vi "Load Tdms Wfm By Index.vi"(8 "error in (no error)":errorcluster, 10 "Read From":i32, 11 "file path":path) -> (0 "error out":errorcluster, 3 "Waveform":waveform(dbl)(graph))   [LabVIEW 2025, in "TDMS Waveform Creator.lvclass"]
uses:
  TDMS Waveform Creator.lvclass
  TDMS Waveform Creator.lvclass/TDMS Waveform Creator.ctl
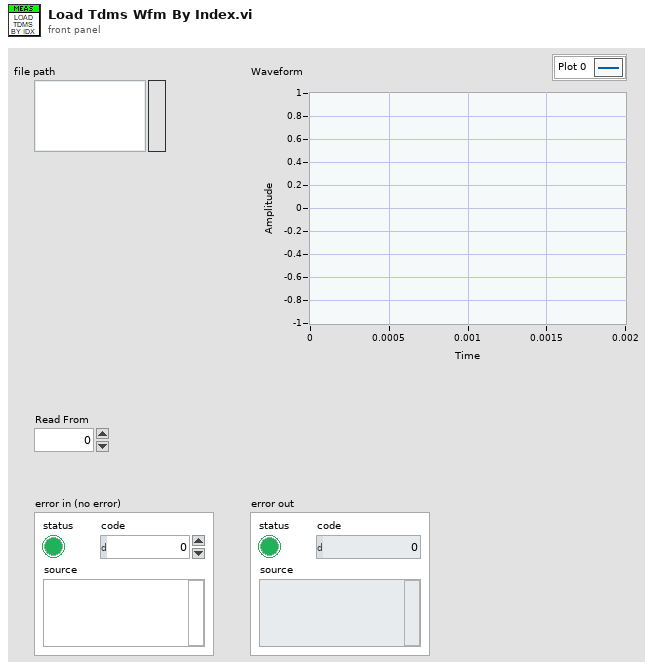
[diagram p1: front panel]
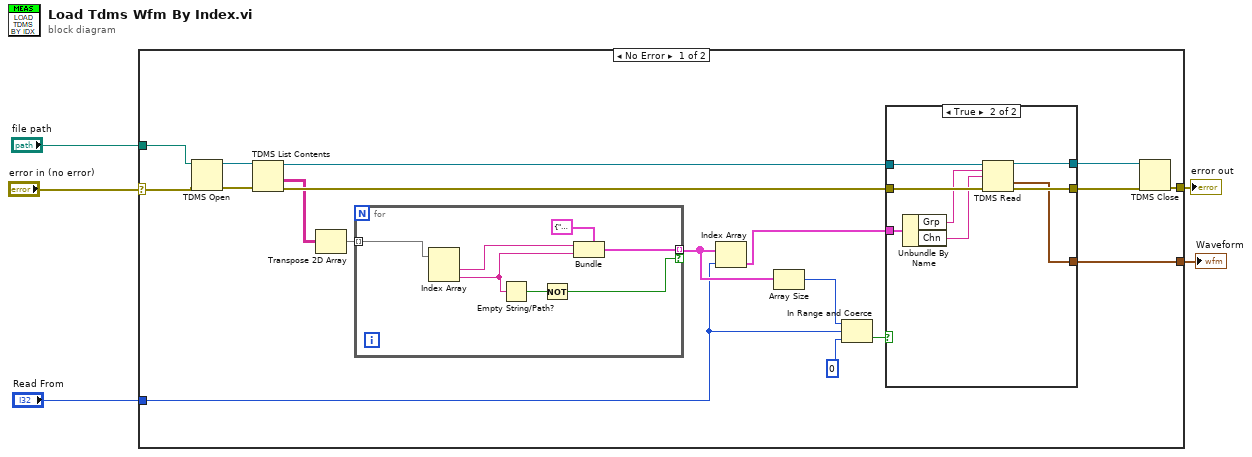
[diagram p0: block diagram]
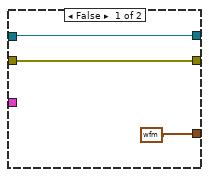
[diagram p2: hidden frame]
diagram:
  n1 = case shown="No Error" "error in (no error)" {
    selector: "error in (no error)" -> [w7 w42]
    tunnel: "file path" -> [w23 _]
    tunnel: [w13 _] -> w4
    tunnel: "Read From" -> [w9 _]
    tunnel: [w6 w42] -> w1
    frame No Error {
      n2 = TDMS Open(8:w7, 11:w23) -> (0:w22:errorcluster, 3:w21:refnum<k34>)  [unwired: 5 in]
      n3 = TDMS List Contents(4:w22, 7:w21) -> (0:w20:errorcluster, 1:w19:string[][], 3:w16:refnum<k34>)  [unwired: 1 in, 1 out]
      n4 = Transpose 2D Array(2D array=w19) -> (transposed array=w18:string[][])
      n5 = for {
        tunnel: w18 -> [w41] mode=indexing
        tunnel: [w36] -> w12 mode=indexing if=w35
        n6 = Index Array(array=w41) -> (element #1=w38:string, element #2=w39:string)  [unwired: 2 in]
        n7 = Empty String/Path?(string/path=w39) -> (empty?=w40:bool)
        n8 = Not(x=w40) -> (.not. x?=w35:bool)
        n9 = Bundle(cluster=cluster{"Grp":string, "Chn":string} {"Grp"="", "Chn"=""} ("output cluster"), "Grp"=w38, "Chn"=w39) -> (w36:cluster{"Grp":string, "Chn":string})
      }
      n10 = Index Array(array=w12, index=w9) -> (element=w14:cluster{"Grp":string, "Chn":string})
      n11 = Array Size(array=w12) -> (size(s)=w11:i32)
      n12 = In Range and Coerce(upper limit=w11, x=w9, lower limit=0) -> (In Range?=w8:bool)  [unwired: 1 out]
      n13 = case shown="True" w8 {
        tunnel: w20 -> [w25 w34]
        tunnel: [w25 w33] -> w17
        tunnel: w16 -> [w26 w32]
        tunnel: [w26 w31] -> w15
        tunnel: w14 -> [_ w30]
        tunnel: [waveform(dbl) {"t0"=timestamp(0 s since 1904-01-01), "dt"=1.0, "Y"=[]} w27] -> w13
        frame False {
        }
        frame True {
          n14 = Unbundle By Name(w30) -> ("Grp"=w29:string, "Chn"=w28:string)
          n15 = TDMS Read(0:w32, 5:w29, 7:w28, 11:w34) -> (4:w31:refnum<k34>, 10:w27:waveform(dbl), 15:w33:errorcluster)  [unwired: 4 in, 3 out]
        }
      }
      n16 = TDMS Close(8:w17, 11:w15) -> (0:w6:errorcluster)  [unwired: 1 out]
    }
    frame Error {
    }
  }
  "Waveform" <- w4
  "error out" <- w1
